vi "test harness_FXP_A_times_x.vi"() -> ()   [LabVIEW 2017, in "FXP_observer_TestCase.lvclass"]
uses:
  FXP_observer_TestCase.lvclass
  fpga_VIs/fpga_subVIs_ssxy/fixed-point-ss/typeDefs/x_vec_scalar.ctl
  C:/Program Files (x86)/National Instruments/LabVIEW 2017/vi.lib/addons/_JKI Toolkits/VI Tester/TestCase.llb/TestCase.lvclass
  <vilib>/rvi/DesktopExecutionNode/Execution/niFpgaDEN_Execute.vi
  <vilib>/rvi/DesktopExecutionNode/DesktopExecutionNode.xnode
  <userlib>/_VITAC/VITAC.lvlib
panel:
  out "error out":errorcluster
  out "TestCase out":refnum<class "FXP_observer_TestCase.lvclass">
  in  "TestCase in":refnum<class "FXP_observer_TestCase.lvclass">
  in  "error in (no error)":errorcluster
  out "X_vec":T1[](array[typedef])
  out "xk_1_1":fxp<+/-,32,6>[](array[numeric])
  out "A*x":fxp<+/-,32,13>[](array[numeric])
  out "A*x (expected)":fxp<+/-,64,12>[](array[numeric])
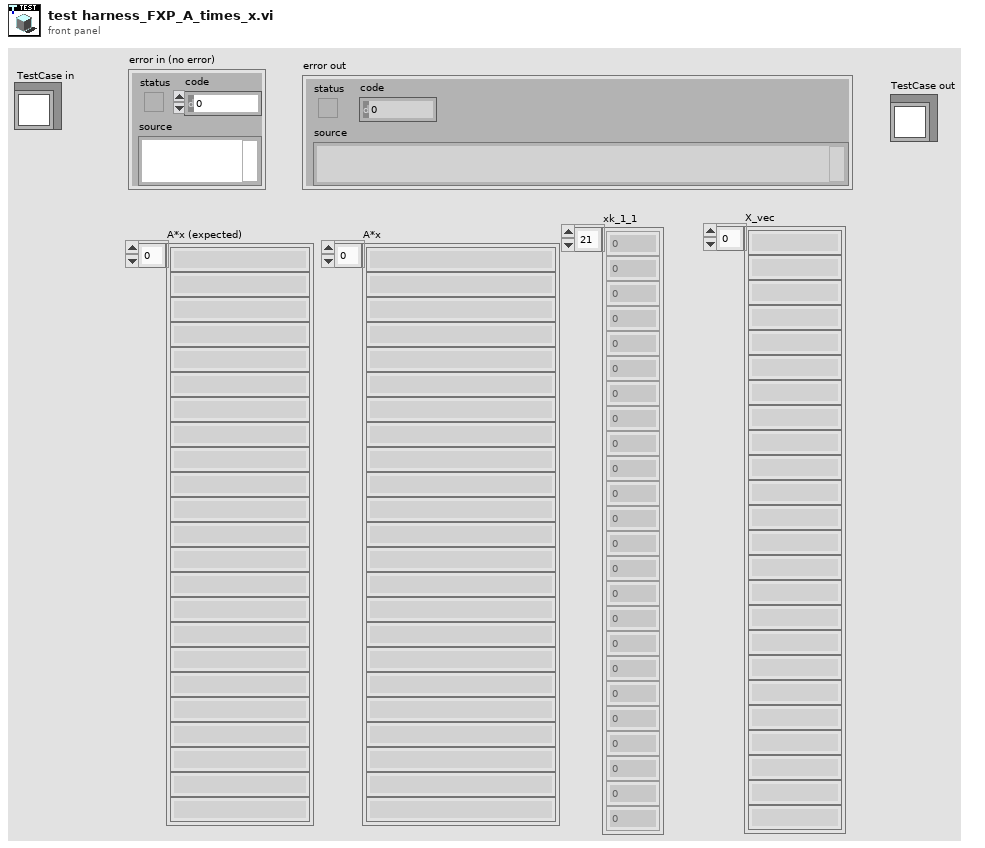
[diagram p1: front panel]
types:
  T1 = typedef "x_vec_scalar.ctl" = fxp<+/-,32,6>
  T2 = typedef "UT_matrix_data.ctl" = cluster{"Bz":T3[], "Ldist":T4[], "Kz":T5[], "Nx":T6[], "Ax_col":T7[], "X_vec":T1[], "Cz":T8[]}
  T3 = typedef "Bz_vec_scalar.ctl" = fxp<+/-,32,3>
  T4 = typedef "Lz_vec_scalar.ctl" = fxp<+/-,32,3>
  T5 = typedef "Kz_vec_scalar.ctl" = fxp<+/-,32,10>
  T6 = typedef "Nx_vec_scalar.ctl" = fxp<+/-,32,2>
  T7 = typedef "Az_vec_scalar.ctl" = fxp<+/-,32,7>
  T8 = typedef "Cz_vec_scalar.ctl" = fxp<+/-,32,4>
  T9 = typedef "x_vec_type.ctl" = fxp<+/-,32,6>[]
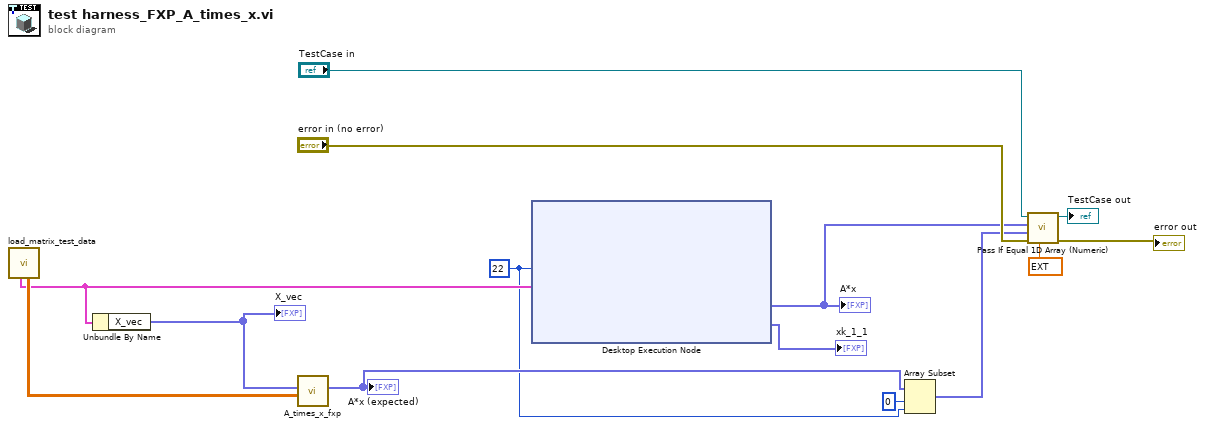
[diagram p0: block diagram]
diagram:
  w2 = u8 22 ("NS + 1")
  n1 = call "load_matrix_test_data.vi"() -> ("A_mat"=w14:dbl[][], "output cluster"=w12:T2)  [unwired: 4 in, 6 out]
  n2 = Unbundle By Name(w12) -> ("X_vec"=w13:T1[])
  "X_vec" <- w13
  n3 = call "A_times_x_fxp.vi"("Az_mat in"=w14, "x_vec"=w13) -> ("A*x"=w4:T9)  [unwired: 8 in, 1 out]
  "A*x (expected)" <- w4
  n4 = xnode "Desktop Execution Node"("NS"=w2, "matrix data"=w12) -> ("A*x"=w5:fxp<+/-,32,13>[], "xk_1_1"=→"xk_1_1":fxp<+/-,32,6>[])  [unwired: 1 in, 1 out]
  "A*x" <- w5
  n5 = Array Subset(array=w4, index=0, length=w2) -> (w1:fxp<+/-,32,6>[])
  n6 = call <userlib>:"Pass If Equal 1D Array (Numeric).vi"("delta (optional)"=ext 0.00001, "error in (no error)"="error in (no error)", "actual"=w1, "expected"=w5, "TestCase in"="TestCase in") -> ("error out"=→"error out":errorcluster, "TestCase out"=→"TestCase out":refnum<class "FXP_observer_TestCase.lvclass">)  [unwired: 5 in]
